vi "Tetra_Set-Freq.vi"(0 "COMPORT":refnum<visa-resource-name>="COM4", 5 "error in (no error)":errorcluster, 7 "Freq":dbl=20.0, 8 "delay after set(ms)":u32, 9 "Freq Units":u16(ring)=1 items=["MHz", "GHz"], 11 "Open Ser(t)":bool, 13 "Close Ser(t)":bool) -> (10 "Success":bool=TRUE, 12 "output":string="freq 20000\r\n>", 14 "comport":refnum<visa-resource-name>="COM4", 19 "error out":errorcluster)   [LabVIEW 2018]
uses:
  <vilib>/Utility/error.llb/Error Cluster From Error Code.vi
  <vilib>/ErrorRing/Error Ring.xnode
panel:
  out "In Range?":bool=TRUE
  # "Must write : wr reg 0x04 1032\nprior to use"
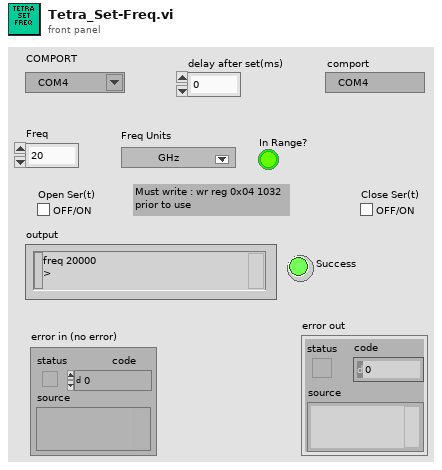
[diagram p1: front panel]
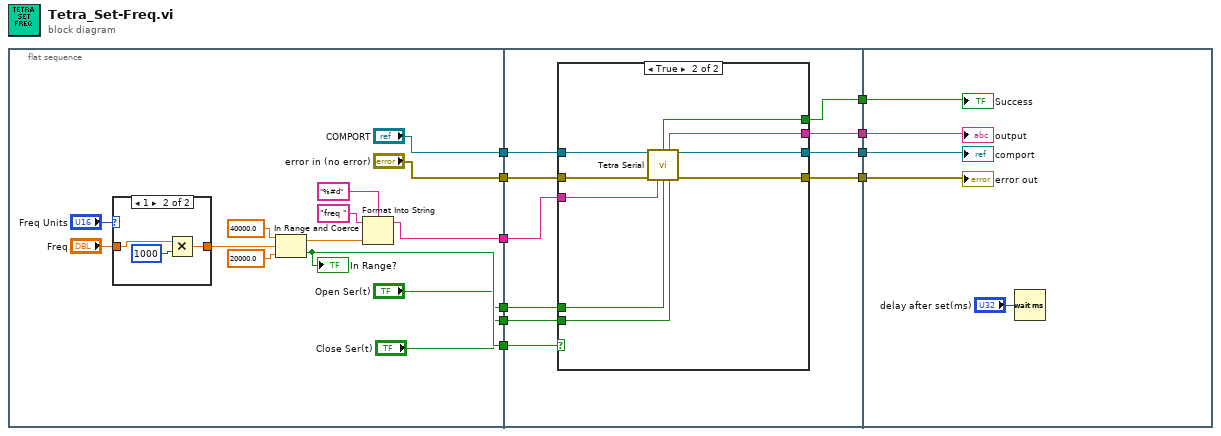
[diagram p0: block diagram]
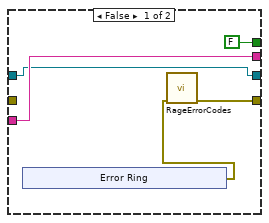
[diagram p3: hidden frame]
diagram:
  n1 = flat-sequence {
    tunnel: ["error in (no error)"] -> w6
    tunnel: ["COMPORT"] -> w5
    tunnel: ["Open Ser(t)"] -> w4
    tunnel: ["Close Ser(t)"] -> w3
    tunnel: [w15] -> w2
    tunnel: [w16] -> w1
    tunnel: [w38] -> w10
    tunnel: [w35] -> w9
    tunnel: [w32] -> w8
    tunnel: [w31] -> w7
    tunnel: w6 -> [w37]
    tunnel: w5 -> [w36]
    tunnel: w4 -> [w34]
    tunnel: w3 -> [w33]
    tunnel: w2 -> [w30]
    tunnel: w1 -> [w29]
    tunnel: w10 -> [w58]
    tunnel: w9 -> [w59]
    tunnel: w8 -> [w60]
    tunnel: w7 -> [w61]
    frame #0 {
      n2 = case shown="1" "Freq Units" {
        tunnel: "Freq" -> [w25 w28]
        tunnel: [w25 w27] -> w23
        frame 0, Default {
        }
        frame 1 {
          n3 = Multiply(x=w28, y=1000) -> (x*y=w27:dbl)
        }
      }
      n4 = In Range and Coerce(upper limit=40000.0, x=w23, lower limit=20000.0) -> (coerced(x)=w24:dbl, In Range?=w16:bool)
      "In Range?" <- w16
      n5 = Format Into String(format string="%#d", initial string="freq " ("string"), w24) -> (resulting string=w15:string)  [unwired: 1 in, 1 out]
    }
    frame #1 {
      n6 = case shown="True" w29 {
        tunnel: [w43 w56] -> w38
        tunnel: w37 -> [_ w55]
        tunnel: w36 -> [w41 w54]
        tunnel: [w41 w53] -> w35
        tunnel: w34 -> [_ w52]
        tunnel: w33 -> [_ w51]
        tunnel: [w42 w50] -> w32
        tunnel: [FALSE ("Success") w49] -> w31
        tunnel: w30 -> [w42 w48]
        frame False {
          n7 = xnode "Error Ring"() -> ("error out"=w39:errorcluster)
          n8 = call "RageErrorCodes.vi"("error in"=w39) -> ("error out"=w43:errorcluster)  [unwired: 8 in, 2 out]
        }
        frame True {
          n9 = call "Tetra Serial.vi"("COMPORT"=w54, "error in (no error)"=w55, "Command"=w48, "Open Ser(t)"=w52, "Close Ser(t)"=w51) -> ("Success"=w49:bool, "output"=w50:string, "comport"=w53:refnum<visa-resource-name>, "error out"=w56:errorcluster)  [unwired: 6 in, 1 out]
        }
      }
    }
    frame #2 {
      n10 = Wait (ms)(milliseconds to wait="delay after set(ms)") -> ()  [unwired: 1 out]
      "error out" <- w58
      "comport" <- w59
      "output" <- w60
      "Success" <- w61
    }
  }
